vi "fileIO.vi"(8 "file path (dialog if empty)":path) -> (0 "Axial inc (mm)":dbl, 1 "yPosFin (mm)":dbl, 2 "Lateral inc (mm)":dbl, 3 "zPosFin (mm)":dbl, 4 "yPosInit (mm)":dbl, 5 "zPosInit (mm)":dbl, 6 "xPosFin (mm)":dbl, 7 "xPosInit (mm)":dbl)   [LabVIEW 2015]
uses:
  <vilib>/Utility/file.llb/Read Delimited Spreadsheet (DBL).vi
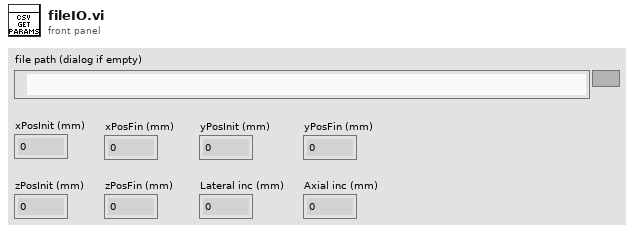
[diagram p1: front panel]
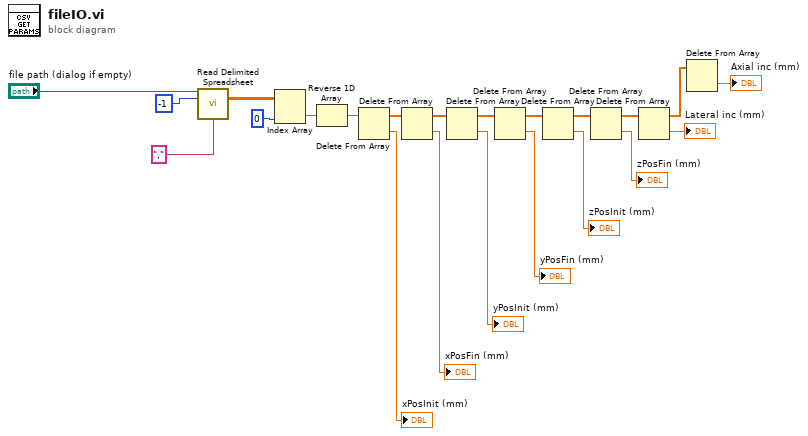
[diagram p0: block diagram]
diagram:
  n1 = call-poly <vilib>:"Read Delimited Spreadsheet.vi"("file path (dialog if empty)"="file path (dialog if empty)", "number of rows (all:-1)"=-1, "delimiter (\\t)"="," ("delimiter (\\t)")) -> ("all rows"=w19:dbl[][])  [unwired: 7 in, 5 out]
  n2 = Index Array(array=w19, index (col)=0 ("disabled index (col)")) -> (element=w17:dbl[])  [unwired: 1 in]
  n3 = Reverse 1D Array(array=w17) -> (reversed array=w16:dbl[])
  n4 = Delete From Array(array=w16) -> (deleted portion=→"xPosInit (mm)":dbl, array with subset deleted=w14:dbl[])  [unwired: 2 in]
  n5 = Delete From Array(array=w14) -> (deleted portion=→"xPosFin (mm)":dbl, array with subset deleted=w12:dbl[])  [unwired: 2 in]
  n6 = Delete From Array(array=w12) -> (deleted portion=→"yPosInit (mm)":dbl, array with subset deleted=w10:dbl[])  [unwired: 2 in]
  n7 = Delete From Array(array=w10) -> (deleted portion=→"yPosFin (mm)":dbl, array with subset deleted=w8:dbl[])  [unwired: 2 in]
  n8 = Delete From Array(array=w8) -> (deleted portion=→"zPosInit (mm)":dbl, array with subset deleted=w6:dbl[])  [unwired: 2 in]
  n9 = Delete From Array(array=w6) -> (deleted portion=→"zPosFin (mm)":dbl, array with subset deleted=w4:dbl[])  [unwired: 2 in]
  n10 = Delete From Array(array=w4) -> (deleted portion=→"Lateral inc (mm)":dbl, array with subset deleted=w2:dbl[])  [unwired: 2 in]
  n11 = Delete From Array(array=w2) -> (deleted portion=→"Axial inc (mm)":dbl)  [unwired: 2 in, 1 out]
